vi "DB - Convert BIT Type.vi"(3 "Boolean":bool, 4 "BIT Type (eg Inactive) (Array)":string[](array[string]), 5 "BIT Type (eg Inactive)":string) -> (0 "BIT (eg Inactive)":string, 1 "Boolean (Array)":bool[](array[boolean]), 2 "Boolean":bool)   [LabVIEW 2020]
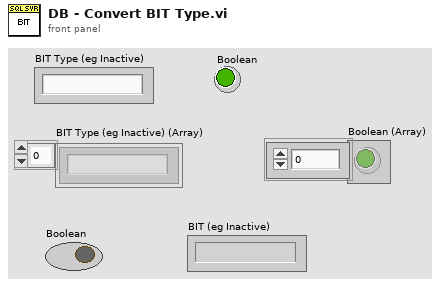
[diagram p1: front panel]
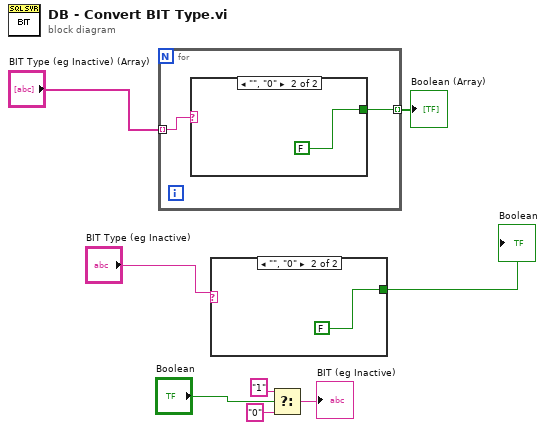
[diagram p0: block diagram]
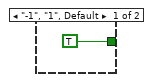
[diagram p2: hidden frame]
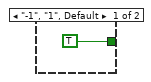
[diagram p3: hidden frame]
diagram:
  n1 = for {
    tunnel: "BIT Type (eg Inactive) (Array)" -> [w10] mode=indexing
    tunnel: [w9] -> w1 mode=indexing
    n2 = case shown="\"\", \"0\"" w10 {
      tunnel: [TRUE FALSE] -> w9
      frame "-1", "1", Default {
      }
      frame "", "0" {
      }
    }
  }
  "Boolean (Array)" <- w1
  n3 = case shown="\"\", \"0\"" "BIT Type (eg Inactive)" {
    tunnel: [TRUE FALSE] -> w6
    frame "-1", "1", Default {
    }
    frame "", "0" {
    }
  }
  "Boolean" <- w6
  n4 = Select(t="1" ("string"), s="Boolean", f="0" ("string")) -> (s? t:f=→"BIT (eg Inactive)":string)
